vi "Write rotPA.vi"(8 "error in (no error)":errorcluster, 10 "rotPA":dbl[unit] min=0.0 max=6.283185307179586, 11 "RotatorPositions in":refnum<class "RotatorPositions.lvclass">) -> (0 "error out":errorcluster, 3 "RotatorPositions out":refnum<class "RotatorPositions.lvclass">)   [LabVIEW 2022 SP3, in "TCSDataDefinitions.lvlib" / "TCSPublicStatus.lvlib" / "PointingPositions.lvlib" / "RotatorPositions.lvclass"]
uses:
  RotatorPositions.lvclass
  RotatorPositions.lvclass/RotatorPositions.ctl
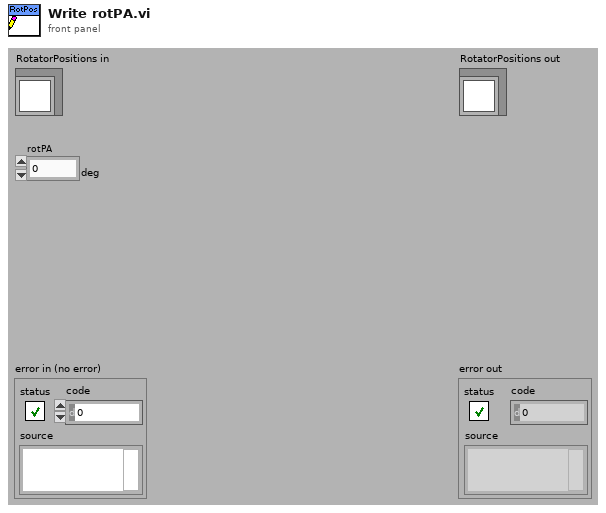
[diagram p1: front panel]
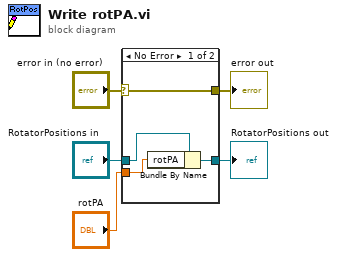
[diagram p0: block diagram]
diagram:
  n1 = case shown="No Error" "error in (no error)" {
    selector: "error in (no error)" -> [w9 w10]
    tunnel: [w9 w10] -> w4
    tunnel: [w7 w11] -> w2
    tunnel: "RotatorPositions in" -> [w8 w11]
    tunnel: "rotPA" -> [w6 _]
    frame No Error {
      n2 = Bundle By Name(cluster=w8, "rotPA"=w6) -> (w7:refnum<class "RotatorPositions.lvclass">)
    }
    frame Error {
    }
  }
  "error out" <- w4
  "RotatorPositions out" <- w2
